vi "Non Stream 4310 DMM.vi"(8 "error in (no error)":errorcluster, 10 "Number of Iterations":i32=10) -> (0 "error out":errorcluster, 1 "4309 Measurements":waveform(dbl)[](array[waveform]), 2 "DMM Measurements":dbl[](array[numeric]))   [LabVIEW 2019]
uses:
  <instrlib>/niDMM/nidmm.llb/niDMM Slope.ctl
  <instrlib>/niDMM/nidmm.llb/niDMM Trigger.ctl
  <instrlib>/niDMM/nidmm.llb/niDMM Resolution in Digits.ctl
  <instrlib>/niDMM/nidmm.llb/niDMM Function.ctl
  <instrlib>/niDMM/nidmm.llb/niDMM Sample Trigger.ctl
  <vilib>/DAQmx/read.llb/DAQmx Read (Analog 1D Wfm NChan NSamp).vi
  <vilib>/DAQmx/create/channels.llb/DAQmx Create Channel (AI-Voltage-Basic).vi
  <vilib>/DAQmx/configure/timing.llb/DAQmx Timing (Sample Clock).vi
  <vilib>/DAQmx/configure/events/hardwareSignals.llb/DAQmx Export Signal (Most Signals).vi
  <instrlib>/niDMM/nidmm.llb/niDMM Configure Measurement Digits.vi
  <vilib>/DAQmx/miscellaneous.llb/DAQmx Fill In Error Info.vi
  <vilib>/Waveform/WDTOps.llb/WDT Append Waveforms DBL.vi
panel:
  in  "Default":waveform(dbl)[](array[waveform])
  in  "Number of Samples":i32=1000
  in  "Sample Rate":dbl=20000.0
  in  "Sample Clock Source":tag="OnboardClock"
  in  "Terminal Configuration":i32(ring)=-1 items=["default"=-1, "RSE"=10083, "NRSE"=10078, "Differential"=10106, "Pseudodifferential"=12529]
  in  "Max Voltage":dbl=5.0
  in  "Min Voltage":dbl=-5.0
  in  "Physical Channel":tag="4309/ai0:7"
  in  "Function":T1
  in  "Resolution in Digits":T2=3.5 items=["3 1/2"=3.5, "4 1/2"=4.5, "5 1/2"=5.5, "6 1/2"=6.5, "7 1/2"=7.5]
  in  "Range":dbl=10.0 format="%.2p"
  in  "Stop":bool
  in  "Trigger Source":T3=enum."TTL 0"
  in  "Slope":T4=enum."Falling Edge"
  in  "Device Name":refnum<k15>="DMM"
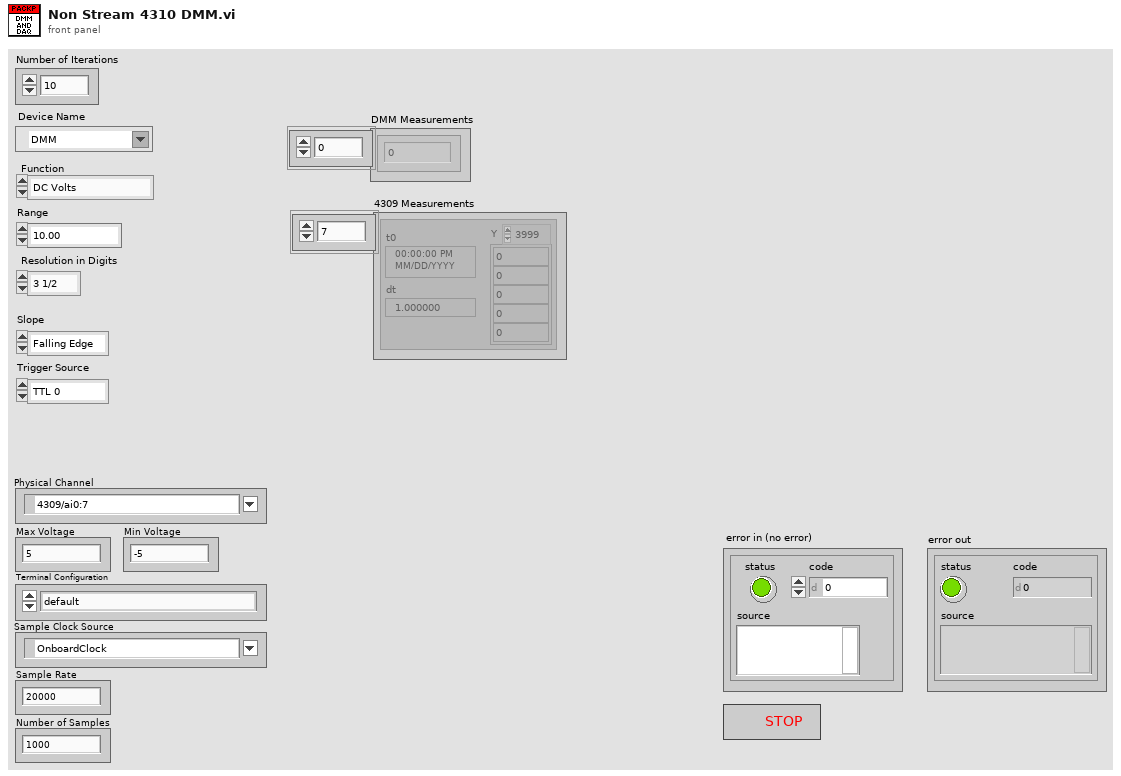
[diagram p1: front panel]
types:
  T1 = typedef "niDMM Function.ctl" = enum16{"DC Volts", "AC Volts", "DC Current", "AC Current", "2-wire Resistance", "4-wire Resistance", "Diode", "Frequency", "Period", "AC Volts DC Coupled", "Capacitance", "Inductance", "Temperature"}
  T2 = typedef "niDMM Resolution in Digits.ctl" = dbl
  T3 = typedef "niDMM Trigger.ctl" = enum16{"Immediate", "External", "TTL 0", "TTL 1", "TTL 2", "TTL 3", "TTL 4", "TTL 5", "TTL 6", "Software", "TTL 7", "PXI Star", "LBR Trig 1", "Aux Trig 1"}
  T4 = typedef "niDMM Slope.ctl" = enum16{"Rising Edge", "Falling Edge"}
  T5 = typedef "niDMM Sample Trigger.ctl" = enum16{"Immediate", "External", "TTL 0", "TTL 1", "TTL 2", "TTL 3", "TTL 4", "TTL 5", "TTL 6", "Interval", "Software", "TTL 7", "PXI Star", "LBR Trig 1", "Aux Trig 1"}
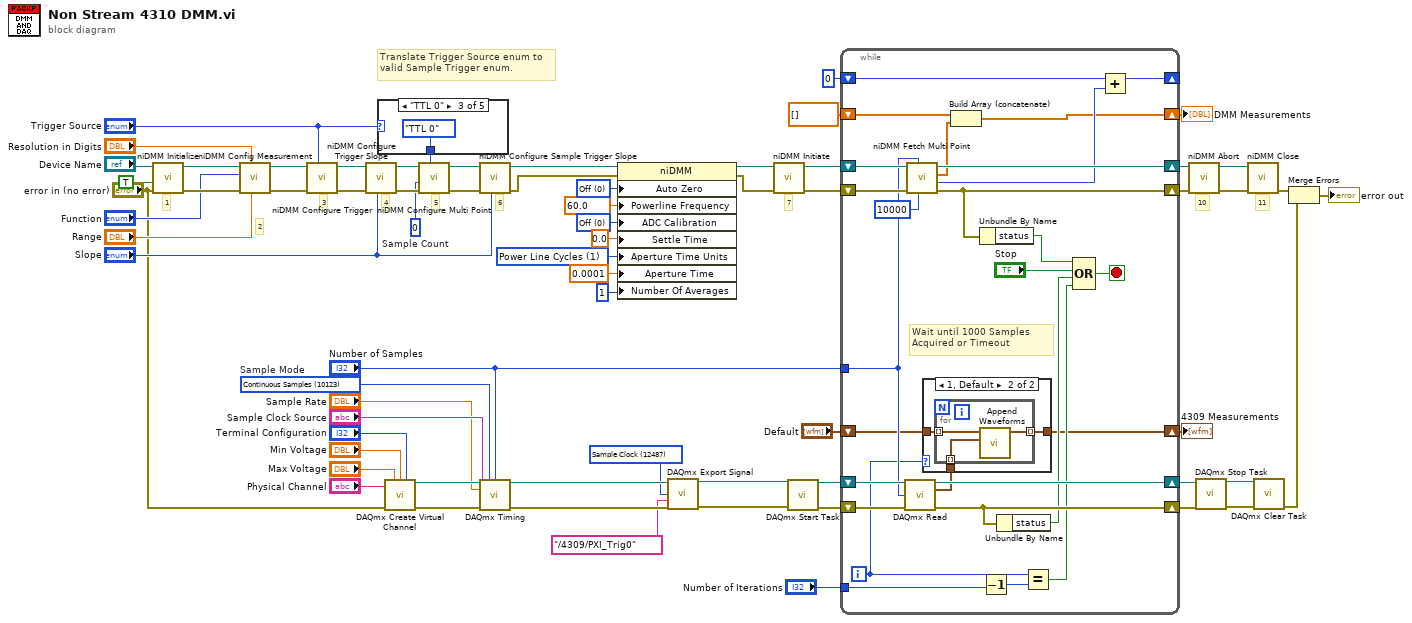
[diagram p0: block diagram]
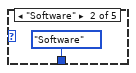
[diagram p4: hidden frame]
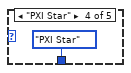
[diagram p5: hidden frame]
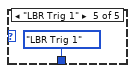
[diagram p6: hidden frame]
diagram:
  w10 = 0 items=["Auto"=-1, "Off"=0, "On"=1, "Once"=2] ("Configuration:Measurement Options:Auto Zero")
  w11 = 60.0 items=["50 Hz"=50.0, "60 Hz"=60.0] ("Configuration:Measurement Options:Powerline Frequency")
  w12 = 0 items=["Auto"=-1, "Off"=0, "On"=1] ("Configuration:Measurement Options:ADC Calibration")
  w14 = 1 items=["Seconds", "Power Line Cycles"] ("Configuration:Advanced:Aperture Time Units")
  w22 = 12487 items=["AI Convert Clock"=12484, "10MHz Reference Clock"=12536, "20MHz Timebase Clock"=12486, "Sample Clock"=12487, "Advance Trigger"=12488, "Reference Trigger"=12490, "Start Trigger"=12491, "Advance Complete Event"=12492, "AI Hold Complete Event"=12493, "Counter Output Event"=12494, "Change Detection Event"=12511, "Watchdog Timer Expired Event"=12512] ("signal")
  w42 = 10123 items=["Finite Samples"=10178, "Continuous Samples"=10123, "Hardware Timed Single Point"=12522]  # Sample Mode
  w51 = 0  # Sample Count
  # "4"
  # "10"
  # "6"
  # "11"
  # "5"
  # "7"
  # "Translate Trigger Source enum to\nvalid Sample Trigger enum."
  # "3"
  # "2"
  # "1"
  n1 = call <instrlib>:"niDMM Initialize.vi"("error in (no error)"="error in (no error)", "Reset"=TRUE, "Instrument Descriptor"="Device Name") -> ("error out"=w67:errorcluster, "instrument handle out"=w68:refnum<k15>)  [unwired: 7 in]
  n2 = call-poly <instrlib>:"niDMM Config Measurement.vi"("Range"="Range", "Resolution in Digits"="Resolution in Digits", "error in (no error)"=w67, "Function"="Function", "instrument handle"=w68) -> ("error out"=w59:errorcluster, "instrument handle out"=w60:refnum<k15>)  [unwired: 5 in]
  n3 = call <instrlib>:"niDMM Configure Trigger.vi"("Trigger Source"="Trigger Source", "error in (no error)"=w59, "instrument handle"=w60) -> ("error out"=w57:errorcluster, "instrument handle out"=w58:refnum<k15>)  [unwired: 7 in]
  n4 = call <instrlib>:"niDMM Configure Trigger Slope.vi"("Slope"="Slope", "error in (no error)"=w57, "instrument handle"=w58) -> ("error out"=w55:errorcluster, "instrument handle out"=w56:refnum<k15>)  [unwired: 7 in]
  n5 = case shown="\"TTL 0\"" "Trigger Source" {
    selector: "Trigger Source" -> [w69 _ _ _ _]
    tunnel: [w69 niDMM_Sample_Trigger."Software" ("Sample Trigger") niDMM_Sample_Trigger."TTL 0" ("Sample Trigger") niDMM_Sample_Trigger."PXI Star" ("Sample Trigger") niDMM_Sample_Trigger."LBR Trig 1" ("Sample Trigger")] -> w46
    frame "Immediate", Default {
    }
    frame "Software" {
    }
    frame "TTL 0" {
    }
    frame "PXI Star" {
    }
    frame "LBR Trig 1" {
    }
  }
  n6 = call-poly <vilib>:"DAQmx Create Virtual Channel.vi"("maximum value"="Max Voltage", "minimum value"="Min Voltage", "input terminal configuration"="Terminal Configuration", "physical channels"="Physical Channel", "error in"="error in (no error)") -> ("task out"=w40:refnum<k21>, "error out"=w41:errorcluster)  [unwired: 9 in]
  n7 = call <instrlib>:"niDMM Configure Multi Point.vi"("Sample Trigger"=w46, "error in (no error)"=w55, "Sample Count"=w51, "instrument handle"=w56) -> ("error out"=w53:errorcluster, "instrument handle out"=w54:refnum<k15>)  [unwired: 6 in]
  n8 = call <instrlib>:"niDMM Configure Sample Trigger Slope.vi"("Slope"="Slope", "error in (no error)"=w53, "instrument handle"=w54) -> ("error out"=w18:errorcluster, "instrument handle out"=w45:refnum<k15>)  [unwired: 7 in]
  n9 = call-poly <vilib>:"DAQmx Timing.vi"("task/channels in"=w40, "sample mode"=w42, "samples per channel"="Number of Samples", "rate"="Sample Rate", "source"="Sample Clock Source", "error in"=w41) -> ("task out"=w26:refnum<k21>, "error out"=w24:errorcluster)  [unwired: 8 in]
  n10 = property class="niDMM"(reference=w45, error in=w18, "Auto Zero"=w10, "Powerline Frequency"=w11, "ADC Calibration"=w12, "Settle Time"=0.0 ("Configuration:Advanced:Settle Time"), "Aperture Time Units"=w14, "Aperture Time"=0.0001 ("Configuration:Advanced:Aperture Time"), "Number Of Averages"=1 ("Configuration:Advanced:Number Of Averages")) -> (reference out=w19:refnum<k15>, error out=w17:errorcluster)
  n11 = call-poly <vilib>:"DAQmx Export Signal.vi"("task/channels in"=w26, "signal"=w22, "output terminal"=tag "/4309/PXI_Trig0", "error in"=w24) -> ("task out"=w25:refnum<k21>, "error out"=w23:errorcluster)  [unwired: 10 in]
  n12 = call <instrlib>:"niDMM Initiate.vi"("error in (no error)"=w17, "instrument handle"=w19) -> ("error out"=w66:errorcluster, "instrument handle out"=w65:refnum<k15>)  [unwired: 8 in]
  n13 = call <vilib>:"DAQmx Start Task.vi"("task/channels in"=w25, "error in"=w23) -> ("task out"=w39:refnum<k21>, "error out"=w38:errorcluster)  [unwired: 12 in]
  n14 = while {
    tunnel: "Number of Samples" -> [w85]
    shift-right: [w100] -> w49
    shift-left: w66 -> [w94]
    shift-right: [w99] -> w48
    shift-left: w65 -> [w93]
    shift-right: [w98] -> w30
    shift-left: w39 -> [w87]
    shift-right: [w97] -> w29
    shift-left: w38 -> [w86]
    shift-right: [w84] -> _
    shift-left: 0 ("Actual Number") -> [w90]
    shift-right: [w81] -> w4
    shift-left: dbl[] [] ("Measurements") -> [w83]
    shift-right: [w76] -> w3
    shift-left: "Default" -> [w77]
    tunnel: "Number of Iterations" -> [w74]
    i -> [w79]
    stop <- w91 stop-if-true
    # "Wait until 1000 Samples Acquired or Timeout"
    n15 = call-poly <vilib>:"DAQmx Read.vi"("task/channels in"=w87, "number of samples per channel"=w85, "error in"=w86) -> ("task out"=w98:refnum<k21>, "data"=w78:waveform(dbl)[], "error out"=w97:errorcluster)  [unwired: 10 in]
    n16 = call <instrlib>:"niDMM Fetch Multi Point.vi"("Maximum Time (msec)"=10000, "Number to Fetch"=w85, "error in (no error)"=w94, "instrument handle"=w93) -> ("error out"=w100:errorcluster, "Actual Number"=w89:i32, "Measurements"=w82:dbl[], "instrument handle out"=w99:refnum<k15>)  [unwired: 4 in]
    n17 = case shown="1, Default" w79 {
      tunnel: w78 -> [w101 w104]
      tunnel: w77 -> [_ w102]
      tunnel: [w101 w103] -> w76
      frame 0 {
      }
      frame 1, Default {
        n18 = for {
          tunnel: w104 -> [w106] mode=indexing
          tunnel: [w105] -> w103 mode=indexing
          tunnel: w102 -> [w107] mode=indexing
          n19 = call-poly <vilib>:"Append Waveforms.vi"("waveform B"=w106, "waveform A"=w107) -> ("waveform out"=w105:waveform(dbl))  [unwired: 8 in, 1 out]
        }
      }
    }
    n20 = Build Array (concatenate)(w83, w82) -> (w81:dbl[])
    n21 = Unbundle By Name(w100) -> ("status"=w96:bool)
    n22 = Decrement(x=w74) -> (x-1=w75:i32)
    n23 = Unbundle By Name(w97) -> ("status"=w92:bool)
    n24 = Equal?(x=w79, y=w75) -> (x = y?=w88:bool)
    n25 = Compound Arithmetic op=OR(w96, "Stop", w92, w88) -> (w91:bool)
    n26 = Add(x=w90, y=w89) -> (x+y=w84:i32)
  }
  "DMM Measurements" <- w4
  "4309 Measurements" <- w3
  n27 = call <instrlib>:"niDMM Abort.vi"("error in (no error)"=w49, "instrument handle"=w48) -> ("error out"=w63:errorcluster, "instrument handle out"=w64:refnum<k15>)  [unwired: 8 in]
  n28 = call <vilib>:"DAQmx Stop Task.vi"("task/channels in"=w30, "error in"=w29) -> ("task out"=w27:refnum<k21>, "error out"=w28:errorcluster)  [unwired: 12 in]
  n29 = call <instrlib>:"niDMM Close.vi"("error in (no error)"=w63, "instrument handle"=w64) -> ("error out"=w8:errorcluster)  [unwired: 9 in]
  n30 = call <vilib>:"DAQmx Clear Task.vi"("task in"=w27, "error in"=w28) -> ("error out"=w7:errorcluster)  [unwired: 13 in]
  n31 = Merge Errors(w8, w7) -> (→"error out":errorcluster)
